vi "#3.vi"(0 "System no.":i32=1 min=1 max=4 step=1, 5 "error in":errorcluster) -> (14 "Position":dbl[](array[numeric]) format="%.6f", 15 "Queried axes out":string[](array[string]), 19 "error out":errorcluster)   [LabVIEW 2020]
doc: "Returns position information. Command is equivalent to POS?.\n\nC-887, F-206: Only for GCS syntax version = GCS 2.0 or higher (check with CSV?.vi. If CSV?.vi is not supported, syntax version is GCS 1.0).\n\nM-8X0: Check HLP?/HELP anwer to find out if #3 is supported. For GCS syntax version = GCS 1.0 (Check with CSV?.vi. If CSV?.vi is not supported, syntax version is GCS 1.0), reports target position of hexapod axes X, Y, Z, U, V, W. Only for controllers based on C-842.80.\nFor GCS syntax version = GCS 2.0 or higher, reports current position."
panel:
  # "Returns position information. Command is equivalent to POS?."
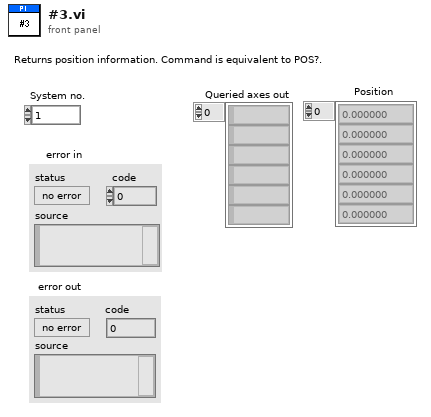
[diagram p1: front panel]
types:
  T1 = enum16{"Disable error check", "Force error check", "Use global settings"}
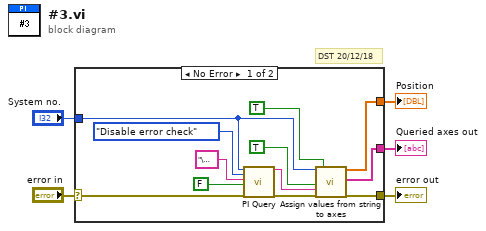
[diagram p0: block diagram]
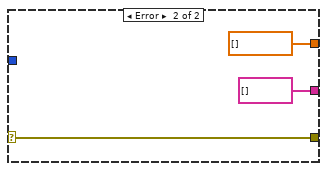
[diagram p2: hidden frame]
diagram:
  # "DST 20/12/18"
  n1 = case shown="No Error" "error in" {
    selector: "error in" -> [w7 w18]
    tunnel: [w16 dbl[] [] ("Values")] -> w5
    tunnel: [w12 w18] -> w4
    tunnel: "System no." -> [w15 _]
    tunnel: [w11 string[] [] ("Queried axes out")] -> w2
    frame No Error {
      n2 = call "PI Query.vi"("System no."=w15, "Error check settings"=T1."Disable error check", "String to send"="\u0003", "Attach termination char.?"=FALSE ("Attach Linefeed?"), "error in"=w7) -> ("String read"=w9:string, "error out"=w8:errorcluster)  [unwired: 2 in, 11 out]
      n3 = call "Assign values from string to axes.vi"("System no."=w15, "All axes queried?"=TRUE, "Input String"=w9, "error in"=w8, "Axes related?"=TRUE) -> ("Values"=w16:dbl[], "Queried axes out"=w11:string[], "error out"=w12:errorcluster)  [unwired: 4 in, 8 out]
    }
    frame Error {
    }
  }
  "error out" <- w4
  "Position" <- w5
  "Queried axes out" <- w2
